vi "structure_tests.vi"() -> ()   [LabVIEW 2010]
panel:
  in  "do some event":bool
  out "Numeric":dbl
  in  "stop little loop":bool
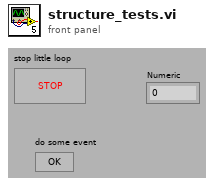
[diagram p1: front panel]
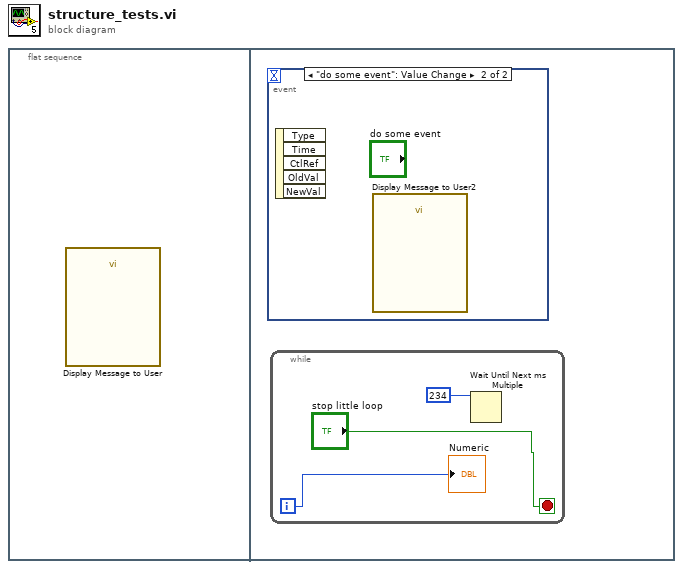
[diagram p0: block diagram]
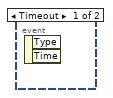
[diagram p2: hidden frame]
diagram:
  n1 = flat-sequence {
    frame #0 {
      n2 = call "Display Message to User"() -> ()  [unwired: 10 in, 2 out]
    }
    frame #1 {
      n3 = event shown="[1] \"do some event\": Value Change" {
        selector: _ -> [_ _]
        dyn-events: _ -> [_ _]
        timeout: _ -> [_ _]
        event Timeout {
          n4 = event-data() -> ()  [unwired: 1 in, 2 out]
        }
        event "do some event": Value Change {
          n5 = event-data() -> ()  [unwired: 1 in, 5 out]
          n6 = call "Display Message to User2"() -> ()  [unwired: 10 in, 2 out]
        }
      }
      n7 = while {
        i -> [w3]
        stop <- "stop little loop" stop-if-true
        n8 = Wait Until Next ms Multiple(millisecond multiple=234) -> ()  [unwired: 1 out]
        "Numeric" <- w3
      }
    }
  }
